vi "1_VisualAD_Train_Eval.vi"(0 "NNFE_Paths":T11={"CFG"=path "D:/Ngene/Projects_SVN/AD/Projects/2025/2025_04_09_VAD_RT_NIConnect/VAD_Host_Train_v1.0/NNFE/RN18_2/RN18_2_bnMerge.cfg", "BIN"=path "D:/Ngene/Projects_SVN/AD/Projects/2025/2025_04_09_VAD_RT_NIConnect/VAD_Host_Train_v1.0/NNFE/RN18_2/RN18_2_bnMerge.bin"}, 1 "Dest. Path":path=path "D:/Working/Cards_3Clubs", 2 "Dataset_Path(Train)":path=path "D:/DNN/_AD/_from_Customers/2025_04_12_NIConnect_3Clubs/1_Dataset/00_Orig/3Clubs/Train", 3 "Dataset_Path(Validation)":path=path "D:/DNN/_AD/_from_Customers/2025_04_12_NIConnect_3Clubs/1_Dataset/00_Orig/3Clubs/Test", 4 "Ground_Truth_Folder_Path":path, 5 "error in":errorcluster, 6 "NNFE_CFG":T7={"Name"="Cards_v2", "Layer_Selection_By"=enum."Layer_Idx", "Feature_Layers"={"[LayerID, PatchSize]"=[{"Layer_ID"=15, "Patch_Size"=5}]}, "Interpolation_Type"=enum."Bi-Linear"}, 7 "Dim_Reduction":T5={"Method"=enum."None", "Target_Dim"=-1, "Seed"=42}, 8 "NNPC_Setup":T13={"Input_Dims"={"C"=3, "H"=256, "W"=256}, "mBatch"=1, "Device"=enum."GPU", "GPU Id"=0}, 9 "Coreset_Params":T12={"CoreSet_Size"=1200.0, "Start_idx"=3}) -> (11 "MemBank Size":i32=1200, 13 "dT_Total":dbl=9.57656679999991 format="%.2p", 14 "NNPC_Paths":T11={"CFG"=path "D:/Working/Cards_3Clubs/NNPC_Cards_v2__25_04_14__17_27_09/NNPC_Cards_v2.cfg", "BIN"=path "D:/Working/Cards_3Clubs/NNPC_Cards_v2__25_04_14__17_27_09/NNPC_Cards_v2.bin"}, 15 "Evaluation_Metrics":T1={"Evaluation_Metrics(Pixel)"={"Scores(Good)"={"X Values"=[0.5210284759104251, 0.6102966575324535, 0.6995648391544819, 0.7888330207765102, 0.8781012023985386, 0.9673693840205669, 1.0566375656425953, 1.1459057472646235, 1.2351739288866521, 1.3244421105086803, 1.4137102921307085, 1.5029784737527372, 1.5922466553747654, 1.6815148369967936, 1.770783018618822, 1.8600512002408505, 1.9493193818628787, 2.0385875634849073, 2.1278557451069355, 2.2171239267289637, 2.306392108350992, 2.39566028997302, 2.484928471595049, 2.5741966532170775, 2.6634648348391057, 2.752733016461134, 2.842001198083162, 2.9312693797051903, 3.020537561327219, 3.109805742949247, 3.199073924571276, 3.288342106193304, 3.3776102878153322, 3.4668784694373604, 3.556146651059389, 3.6454148326814173, 3.734683014303446, 3.823951195925474, 3.9132193775475024, 4.002487559169531, 4.091755740791559, 4.181023922413587, 4.270292104035615, 4.359560285657643, 4.4488284672796725, 4.538096648901701, 4.627364830523729, 4.716633012145758, 4.805901193767786, 4.8951693753898144, 4.984437557011843, 5.073705738633871, 5.162973920255899, 5.252242101877927, 5.3415102834999555, 5.430778465121985, 5.520046646744013, 5.609314828366041, 5.698583009988069, 5.787851191610097, 5.8771193732321265, 5.966387554854155, 6.055655736476183, 6.144923918098211, 6.234192099720239, 6.323460281342268, 6.412728462964296, 6.501996644586324, 6.591264826208353, 6.680533007830381, 6.7698011894524095, 6.859069371074438, 6.948337552696466, 7.037605734318495, 7.126873915940523, 7.216142097562551, 7.30541027918458, 7.394678460806608, 7.483946642428636, 7.573214824050664, 7.6624830056726925, 7.751751187294722, 7.84101936891675, 7.930287550538778, 8.019555732160805, 8.108823913782834, 8.198092095404863, 8.287360277026892, 8.37662845864892, 8.465896640270948, 8.555164821892976, 8.644433003515005, 8.733701185137033, 8.822969366759061, 8.91223754838109, 9.001505730003117, 9.090773911625147, 9.180042093247176, 9.269310274869204, 9.358578456491232], "Histogram: h(x)"=[81, 124, 241, 366, 390, 655, 704, 909, 1257, 1569, 2363, 3876, 6095, 6433, 8148, 12170, 15948, 18555, 21356, 24301, 30533, 36030, 36647, 42002, 51965, 62635, 75376, 90060, 106995, 128101, 153148, 178169, 209892, 250937, 293012, 337008, 377469, 414170, 435302, 432424, 396009, 325877, 240699, 146788, 79579, 37092, 14124, 3355, 769, 100, 0, 0, 0, 0, 0, 0, 0, 0, 0, 0, 0, 0, 0, 0, 0, 0, 0, 0, 0, 0, 0, 0, 0, 0, 0, 0, 0, 0, 0, 0, 0, 0, 0, 0, 0, 0, 0, 0, 0, 0, 0, 0, 0, 0, 0, 0, 0, 0, 0, 0]}, "Scores(Bad)"={"X Values"=[0.5210284759104251, 0.6102966575324535, 0.6995648391544819, 0.7888330207765102, 0.8781012023985386, 0.9673693840205669, 1.0566375656425953, 1.1459057472646235, 1.2351739288866521, 1.3244421105086803, 1.4137102921307085, 1.5029784737527372, 1.5922466553747654, 1.6815148369967936, 1.770783018618822, 1.8600512002408505, 1.9493193818628787, 2.0385875634849073, 2.1278557451069355, 2.2171239267289637, 2.306392108350992, 2.39566028997302, 2.484928471595049, 2.5741966532170775, 2.6634648348391057, 2.752733016461134, 2.842001198083162, 2.9312693797051903, 3.020537561327219, 3.109805742949247, 3.199073924571276, 3.288342106193304, 3.3776102878153322, 3.4668784694373604, 3.556146651059389, 3.6454148326814173, 3.734683014303446, 3.823951195925474, 3.9132193775475024, 4.002487559169531, 4.091755740791559, 4.181023922413587, 4.270292104035615, 4.359560285657643, 4.4488284672796725, 4.538096648901701, 4.627364830523729, 4.716633012145758, 4.805901193767786, 4.8951693753898144, 4.984437557011843, 5.073705738633871, 5.162973920255899, 5.252242101877927, 5.3415102834999555, 5.430778465121985, 5.520046646744013, 5.609314828366041, 5.698583009988069, 5.787851191610097, 5.8771193732321265, 5.966387554854155, 6.055655736476183, 6.144923918098211, 6.234192099720239, 6.323460281342268, 6.412728462964296, 6.501996644586324, 6.591264826208353, 6.680533007830381, 6.7698011894524095, 6.859069371074438, 6.948337552696466, 7.037605734318495, 7.126873915940523, 7.216142097562551, 7.30541027918458, 7.394678460806608, 7.483946642428636, 7.573214824050664, 7.6624830056726925, 7.751751187294722, 7.84101936891675, 7.930287550538778, 8.019555732160805, 8.108823913782834, 8.198092095404863, 8.287360277026892, 8.37662845864892, 8.465896640270948, 8.555164821892976, 8.644433003515005, 8.733701185137033, 8.822969366759061, 8.91223754838109, 9.001505730003117, 9.090773911625147, 9.180042093247176, 9.269310274869204, 9.358578456491232], "Histogram: h(x)"=[131, 229, 343, 603, 652, 1004, 1224, 1485, 2177, 2667, 4288, 6774, 8552, 9591, 12914, 16677, 21984, 26086, 28236, 34100, 43533, 49702, 50940, 58577, 72709, 91728, 107407, 123475, 140133, 161571, 190960, 221005, 254784, 296306, 338720, 381955, 420647, 455243, 485230, 496593, 476018, 425984, 353689, 255448, 182116, 134329, 107803, 94493, 86226, 79961, 74940, 70797, 67724, 65255, 63380, 62473, 61758, 60556, 58820, 57829, 56854, 56149, 54719, 53459, 52357, 50751, 48587, 46892, 43031, 39688, 34785, 30380, 26158, 23541, 20915, 18284, 16302, 14200, 11400, 9383, 7280, 5316, 3813, 2689, 1681, 1310, 660, 301, 98, 55, 55, 53, 46, 44, 46, 37, 39, 36, 37, 35]}, "Eval Stats"={"Scores(Good)"={"Min"=0.49286556, "Max"=4.9073877}, "Scores(Bad)"={"Min"=0.4763944, "Max"=9.403213}, "# of Samples(Good)"=5111808, "# of Samples(Bad)"=8192000, "AUROC"=0.6164574, "F1_Max"=0.7621951, "Thrshld(F1_Max)"=0.4763944, "Prec.(F1_Max)"=0.61576355, "Recall(F1_Max)"=1.0, "FPR(F1_Max)"=1.0, "FNR(F1_Max)"=0.0}}, "Evaluation_Metrics(Image)"={"Scores(Good)"={"X Values"=[4.919271998405456, 4.968675293922424, 5.0180785894393924, 5.06748188495636, 5.116885180473328, 5.166288475990296, 5.215691771507263, 5.26509506702423, 5.314498362541199, 5.363901658058166, 5.413304953575134, 5.462708249092103, 5.51211154460907, 5.561514840126037, 5.610918135643006, 5.660321431159973, 5.70972472667694, 5.759128022193909, 5.808531317710877, 5.857934613227844, 5.907337908744813, 5.95674120426178, 6.006144499778747, 6.055547795295716, 6.104951090812683, 6.154354386329651, 6.203757681846619, 6.253160977363587, 6.302564272880554, 6.351967568397521, 6.40137086391449, 6.450774159431457, 6.500177454948425, 6.549580750465394, 6.598984045982361, 6.648387341499328, 6.697790637016297, 6.747193932533264, 6.796597228050231, 6.8460005235672, 6.8954038190841676, 6.944807114601135, 6.994210410118104, 7.043613705635071, 7.093017001152038, 7.142420296669007, 7.191823592185974, 7.2412268877029415, 7.2906301832199105, 7.340033478736878, 7.389436774253845, 7.438840069770813, 7.488243365287781, 7.537646660804748, 7.5870499563217155, 7.6364532518386845, 7.685856547355652, 7.735259842872619, 7.784663138389588, 7.834066433906555, 7.883469729423522, 7.932873024940491, 7.9822763204574585, 8.031679615974426, 8.081082911491393, 8.130486207008362, 8.17988950252533, 8.229292798042298, 8.278696093559265, 8.328099389076232, 8.3775026845932, 8.426905980110169, 8.476309275627138, 8.525712571144105, 8.575115866661072, 8.62451916217804, 8.673922457695006, 8.723325753211975, 8.772729048728943, 8.822132344245912, 8.871535639762879, 8.920938935279846, 8.970342230796813, 9.01974552631378, 9.06914882183075, 9.118552117347718, 9.167955412864686, 9.217358708381653, 9.26676200389862, 9.316165299415587, 9.365568594932556, 9.414971890449525, 9.464375185966492, 9.51377848148346, 9.563181777000427, 9.612585072517394, 9.661988368034363, 9.711391663551332, 9.7607949590683, 9.810198254585266], "Histogram: h(x)"=[3, 4, 10, 14, 14, 14, 9, 4, 3, 2, 0, 0, 0, 1, 0, 0, 0, 0, 0, 0, 0, 0, 0, 0, 0, 0, 0, 0, 0, 0, 0, 0, 0, 0, 0, 0, 0, 0, 0, 0, 0, 0, 0, 0, 0, 0, 0, 0, 0, 0, 0, 0, 0, 0, 0, 0, 0, 0, 0, 0, 0, 0, 0, 0, 0, 0, 0, 0, 0, 0, 0, 0, 0, 0, 0, 0, 0, 0, 0, 0, 0, 0, 0, 0, 0, 0, 0, 0, 0, 0, 0, 0, 0, 0, 0, 0, 0, 0, 0, 0]}, "Scores(Bad)"={"X Values"=[4.919271998405456, 4.968675293922424, 5.0180785894393924, 5.06748188495636, 5.116885180473328, 5.166288475990296, 5.215691771507263, 5.26509506702423, 5.314498362541199, 5.363901658058166, 5.413304953575134, 5.462708249092103, 5.51211154460907, 5.561514840126037, 5.610918135643006, 5.660321431159973, 5.70972472667694, 5.759128022193909, 5.808531317710877, 5.857934613227844, 5.907337908744813, 5.95674120426178, 6.006144499778747, 6.055547795295716, 6.104951090812683, 6.154354386329651, 6.203757681846619, 6.253160977363587, 6.302564272880554, 6.351967568397521, 6.40137086391449, 6.450774159431457, 6.500177454948425, 6.549580750465394, 6.598984045982361, 6.648387341499328, 6.697790637016297, 6.747193932533264, 6.796597228050231, 6.8460005235672, 6.8954038190841676, 6.944807114601135, 6.994210410118104, 7.043613705635071, 7.093017001152038, 7.142420296669007, 7.191823592185974, 7.2412268877029415, 7.2906301832199105, 7.340033478736878, 7.389436774253845, 7.438840069770813, 7.488243365287781, 7.537646660804748, 7.5870499563217155, 7.6364532518386845, 7.685856547355652, 7.735259842872619, 7.784663138389588, 7.834066433906555, 7.883469729423522, 7.932873024940491, 7.9822763204574585, 8.031679615974426, 8.081082911491393, 8.130486207008362, 8.17988950252533, 8.229292798042298, 8.278696093559265, 8.328099389076232, 8.3775026845932, 8.426905980110169, 8.476309275627138, 8.525712571144105, 8.575115866661072, 8.62451916217804, 8.673922457695006, 8.723325753211975, 8.772729048728943, 8.822132344245912, 8.871535639762879, 8.920938935279846, 8.970342230796813, 9.01974552631378, 9.06914882183075, 9.118552117347718, 9.167955412864686, 9.217358708381653, 9.26676200389862, 9.316165299415587, 9.365568594932556, 9.414971890449525, 9.464375185966492, 9.51377848148346, 9.563181777000427, 9.612585072517394, 9.661988368034363, 9.711391663551332, 9.7607949590683, 9.810198254585266], "Histogram: h(x)"=[0, 0, 0, 0, 0, 0, 0, 0, 0, 0, 0, 0, 0, 0, 0, 0, 0, 0, 0, 0, 0, 0, 0, 0, 0, 0, 0, 0, 0, 4, 0, 2, 1, 3, 6, 6, 6, 7, 1, 1, 6, 3, 0, 2, 0, 0, 1, 0, 0, 1, 1, 2, 0, 2, 2, 0, 0, 1, 0, 0, 3, 6, 5, 5, 2, 5, 5, 8, 4, 6, 2, 4, 4, 0, 4, 2, 0, 0, 1, 0, 0, 0, 0, 0, 0, 0, 0, 0, 0, 0, 0, 0, 0, 0, 0, 0, 0, 0, 0, 1]}, "Eval Stats"={"Scores(Good)"={"Min"=4.8945704, "Max"=5.5621405}, "Scores(Bad)"={"Min"=6.3359256, "Max"=9.8349}, "# of Samples(Good)"=78, "# of Samples(Bad)"=125, "AUROC"=1.0, "F1_Max"=1.0, "Thrshld(F1_Max)"=5.5621824, "Prec.(F1_Max)"=1.0, "Recall(F1_Max)"=1.0, "FPR(F1_Max)"=0.0, "FNR(F1_Max)"=0.0}}} {"Evaluation_Metrics(Image)"."Eval Stats"."Recall(F1_Max)" format="%#.5f"; "Evaluation_Metrics(Image)"."Eval Stats"."FPR(F1_Max)" format="%#.5f"; "Evaluation_Metrics(Image)"."Eval Stats"."FNR(F1_Max)" format="%#.5f"; "Evaluation_Metrics(Image)"."Eval Stats"."Prec.(F1_Max)" format="%#.5f"; "Evaluation_Metrics(Image)"."Eval Stats"."F1_Max" format="%#.5f"; "Evaluation_Metrics(Image)"."Eval Stats"."AUROC" format="%#.5f"; "Evaluation_Metrics(Image)"."Eval Stats"."Scores(Bad)"."Min" format="%#_5g"; "Evaluation_Metrics(Image)"."Eval Stats"."Scores(Good)"."Min" format="%#_5g"; "Evaluation_Metrics(Image)"."Eval Stats"."Thrshld(F1_Max)" format="%#_5f"; "Evaluation_Metrics(Pixel)"."Eval Stats"."Recall(F1_Max)" format="%#.5f"; "Evaluation_Metrics(Pixel)"."Eval Stats"."FPR(F1_Max)" format="%#.5f"; "Evaluation_Metrics(Pixel)"."Eval Stats"."FNR(F1_Max)" format="%#.5f"; "Evaluation_Metrics(Pixel)"."Eval Stats"."Prec.(F1_Max)" format="%#.5f"; "Evaluation_Metrics(Pixel)"."Eval Stats"."F1_Max" format="%#.5f"; "Evaluation_Metrics(Pixel)"."Eval Stats"."AUROC" format="%#.5f"; "Evaluation_Metrics(Pixel)"."Eval Stats"."Scores(Bad)"."Min" format="%#_5g"; "Evaluation_Metrics(Pixel)"."Eval Stats"."Scores(Good)"."Min" format="%#_5g"; "Evaluation_Metrics(Pixel)"."Eval Stats"."Thrshld(F1_Max)" format="%#_5f"}, 18 "Dataset Size":i32=285)   [LabVIEW 2020]
uses:
  <vilib>/Ngene/DeepLTK Anomaly Detection Addon/DeepLTK_Anomaly_Detection_Addon/API/Controls/NN_Paths.ctl
  <vilib>/Ngene/DeepLTK Anomaly Detection Addon/DeepLTK_Anomaly_Detection_Addon/API/Controls/NNPC_Setup.ctl
  <vilib>/Ngene/Deep Learning Toolkit/Toolkit/NN_Data/API/NN_Dims(C,H,W).ctl
  <vilib>/Ngene/Deep Learning Toolkit/Toolkit/NN_Network/Controls/NN_Device.ctl
  <vilib>/Ngene/DeepLTK Anomaly Detection Addon/DeepLTK_Anomaly_Detection_Addon/API/Controls/NNPC_Coreset_Params.ctl
  <vilib>/Ngene/DeepLTK Anomaly Detection Addon/DeepLTK_Anomaly_Detection_Addon/API/Controls/NNFE_CFG.ctl
  <vilib>/Ngene/DeepLTK Anomaly Detection Addon/DeepLTK_Anomaly_Detection_Addon/API/Controls/Layer_Selector.ctl
  <vilib>/Ngene/DeepLTK Anomaly Detection Addon/DeepLTK_Anomaly_Detection_Addon/API/Controls/Feature_Layer_Selector.ctl
  <vilib>/Ngene/DeepLTK Anomaly Detection Addon/DeepLTK_Anomaly_Detection_Addon/API/Controls/Interpolation_Selector.ctl
  <vilib>/Ngene/DeepLTK Anomaly Detection Addon/DeepLTK_Anomaly_Detection_Addon/API/Controls/NNPC_Random_Projection_CFG.ctl
  <vilib>/Ngene/DeepLTK Anomaly Detection Addon/DeepLTK_Anomaly_Detection_Addon/API/Controls/Dim_Reduction_Method.ctl
  <vilib>/Ngene/DeepLTK Anomaly Detection Addon/DeepLTK_Anomaly_Detection_Addon/API/Controls/Evaluation_Metrics(Pixel_Image).ctl
  <vilib>/Ngene/DeepLTK Anomaly Detection Addon/DeepLTK_Anomaly_Detection_Addon/API/Controls/Evaluation_Metrics.ctl
  <vilib>/Ngene/DeepLTK Anomaly Detection Addon/DeepLTK_Anomaly_Detection_Addon/API/Controls/Eval_Results.ctl
  <vilib>/Ngene/DeepLTK Anomaly Detection Addon/DeepLTK_Anomaly_Detection_Addon/API/Controls/MinMax.ctl
  <vilib>/Ngene/DeepLTK Anomaly Detection Addon/DeepLTK_Anomaly_Detection_Addon/API/Controls/NNPC_Save_CFG.ctl
  <vilib>/Ngene/DeepLTK Anomaly Detection Addon/DeepLTK_Anomaly_Detection_Addon/API/Controls/NNPC_PreProcessing_Options.ctl
  <vilib>/Ngene/DeepLTK Anomaly Detection Addon/DeepLTK_Anomaly_Detection_Addon/API/Controls/NNPC_DS_Stats.ctl
  <vilib>/Ngene/DeepLTK Anomaly Detection Addon/DeepLTK_Anomaly_Detection_Addon/API/Controls/Image_Stats_RGB.ctl
  subVIs/Dataset_Reader/Controls/Read_Options.ctl
  <vilib>/Ngene/DeepLTK Anomaly Detection Addon/DeepLTK_Anomaly_Detection_Addon/API/NNPC_Generate_Embedding/NNPC_Generate_Embedding(Dataset).vi
  <vilib>/Ngene/DeepLTK Anomaly Detection Addon/DeepLTK_Anomaly_Detection_Addon/API/NNPC_Predict/NNPC_Predict(Dataset).vi
  <vilib>/Ngene/Deep Learning Toolkit/Toolkit/NN_Data/subVIs/Dataset_Destroy/NN_Dataset_Destroy(In3D_Out3D).vi
  <vilib>/Ngene/Deep Learning Toolkit/Toolkit/Deep_Learning_Toolkit_by_Ngene.lvlib
  <vilib>/Ngene/DeepLTK Anomaly Detection Addon/DeepLTK_Anomaly_Detection_Addon/DeepLTK_Anomaly_Detection_Addon.lvlib
panel:
  out "Feature Size":i32=128
  out "error out":errorcluster
  out "Coreset Min":sgl=5.160844
  out "Coreset Max":sgl=19.46937
  out "dT_Predict":dbl=0.5213928000000578 format="%.2p"
  out "dT_Eval":dbl=3.1058166000000256 format="%.2p"
  out "dT_Read_DS(Test)":dbl=2.2328044000000773 format="%.2p"
  out "dT_Read_DS(Train)":dbl=3.5484586999998555 format="%.2p"
  out "dT_NN_Init":dbl=0.5681460999999217 format="%.2p"
  out "Coreset_Max_Distances":sgl[](graph)=[19.46937, 16.781397, 14.001281, 13.836462, 13.739045, 13.200295, 13.1346245, 12.7480755, 12.133151, 11.688953, 11.562293, 11.521474, 11.431094, 11.274108, 11.229277, 11.169556, 11.083287, 10.935635, 10.858421, 10.807946, 10.589487, 10.50305, 10.480584, 10.4153595, 10.357788, 10.130338, 10.12428, 10.081089, 10.0776615, 9.983067, 9.924832, 9.915435, 9.884131, 9.870699, 9.85285, 9.725132, 9.696888, 9.675768, 9.64603, 9.645999, 9.541911, 9.518525, 9.453406, 9.437411, 9.435752, 9.389733, 9.381479, 9.36939, 9.320507, 9.282261, 9.261716, 9.232438, 9.134313, 9.117022, 9.116268, 9.044784, 9.028286, 9.010026, 8.983074, 8.971089, 8.858672, 8.845759, 8.840825, 8.830351, 8.809639, 8.80413, 8.781888, 8.748896, 8.719765, 8.715809, 8.696731, 8.6775675, 8.667834, 8.641909, 8.6257515, 8.603801, 8.565515, 8.5644455, 8.549131, 8.536594, 8.514139, 8.488552, 8.475194, 8.468653, 8.454728, 8.427404, 8.376778, 8.365597, 8.351924, 8.348353, 8.339942, 8.325125, 8.303677, 8.291491, 8.268808, 8.260227, 8.25838, 8.234027, 8.224351, 8.217981, 8.205, 8.191266, 8.13027, 8.124921, 8.121136, 8.108029, 8.091195, 8.082535, 8.079678, 8.071409, 8.068754, 8.062763, 8.04005, 8.0156765, 7.9833508, 7.9817734, 7.9756866, 7.9674706, 7.955339, 7.954186, 7.9532056, 7.951235, 7.932406, 7.9036345, 7.8951316, 7.894743, 7.884721, 7.8842, 7.861708, 7.843711, 7.8291306, 7.8041654, 7.802609, 7.7963605, 7.7932577, 7.787836, 7.777994, 7.768069, 7.76735, 7.7649727, 7.7557883, 7.742485, 7.72457, 7.720849, 7.720424, 7.7061787, 7.6922684, 7.654444, 7.653362, 7.645953, 7.6325245, 7.623823, 7.6200075, 7.597344, 7.591033, 7.5791984, 7.575896, 7.573134, 7.5683107, 7.567111, 7.5648885, 7.5555177, 7.5493193, 7.5422254, 7.5120873, 7.502437, 7.500528, 7.4817066, 7.477346, 7.4752254, 7.4747458, 7.4741282, 7.4712133, 7.455745, 7.446993, 7.443767, 7.4243193, 7.4176674, 7.416217, 7.4160852, 7.4139676, 7.4089565, 7.4084272, 7.399413, 7.3951864, 7.3940825, 7.3912115, 7.389731, 7.368076, 7.3674774, 7.3668766, 7.363222, 7.3573623, 7.337048, 7.3313246, 7.325255, 7.324968, 7.323693, 7.3220134, 7.3206563, 7.3185635, 7.318065, 7.303977, 7.291284, 7.279843, 7.2771497, 7.2746754, 7.246301, 7.2461243, 7.243245, 7.242394, 7.2367034, 7.2228603, 7.214697, 7.2118196, 7.206732, 7.18588, 7.176505, 7.1760736, 7.1721196, 7.1578617, 7.1497097, 7.146749, 7.1445727, 7.1393065, 7.1373143, 7.136985, 7.1265244, 7.1151376, 7.1098557, 7.107177, 7.089042, 7.087757, 7.086635, 7.0733504, 7.072466, 7.062424, 7.054523, 7.053416, 7.051845, 7.0364347, 7.034743, 7.029583, 7.02008, 7.014531, 7.0104465, 7.0066824, 7.005759, 7.005667, 7.0022926, 6.9957547, 6.994208, 6.987603, 6.984908, 6.978115, 6.9691133, 6.9688706, 6.9617443, 6.9612446, 6.944324, 6.942715, 6.9325075, 6.923096, 6.905236, 6.9001384, 6.899265, 6.8963866, 6.8704596, 6.869638, 6.869458, 6.863222, 6.861132, 6.850164, 6.8474054, 6.8398046, 6.831105, 6.82602, 6.82428, 6.814876, 6.8023686, 6.7976675, 6.7915907, 6.790449, 6.788597, 6.783666, 6.777097, 6.7768, 6.7766695, 6.7756424, 6.7756314, 6.7743025, 6.7706504, 6.769866, 6.7661753, 6.7629337, 6.7596316, 6.7594075, 6.7484965, 6.7453437, 6.7376823, 6.731993, 6.727994, 6.724348, 6.7240124, 6.718407, 6.7123427, 6.7033186, 6.7010183, 6.700698, 6.6960373, 6.692671, 6.6923537, 6.6918955, 6.691252, 6.6697273, 6.665576, 6.665223, 6.660309, 6.6597266, 6.659044, 6.6538057, 6.6527185, 6.6511774, 6.6489587, 6.640832, 6.6406984, 6.6404, 6.636598, 6.629583, 6.6145883, 6.611282, 6.609181, 6.6089616, 6.6086326, 6.6038976, 6.5997596, 6.5987697, 6.590461, 6.5878315, 6.586118, 6.585808, 6.5830593, 6.581154, 6.577355, 6.576863, 6.576478, 6.57616, 6.5730104, 6.5719056, 6.5660796, 6.565064, 6.561449, 6.557769, 6.5516324, 6.5426483, 6.5376134, 6.5357857, 6.5316052, 6.5263653, 6.521498, 6.5108414, 6.5060773, 6.505716, 6.502103, 6.500216, 6.498325, 6.4902883, 6.4879932, 6.4849396, 6.4795256, 6.478878, 6.473216, 6.472332, 6.471974, 6.458823, 6.4584785, 6.458313, 6.4524345, 6.4481573, 6.4459114, 6.444943, 6.441784, 6.435836, 6.435274, 6.433396, 6.4295144, 6.427682, 6.4266396, 6.4229894, 6.4196053, 6.40881, 6.406805, 6.4055495, 6.403603, 6.3955894, 6.389062, 6.377372, 6.3744783, 6.3712792, 6.3692875, 6.368519, 6.3667226, 6.3636675, 6.361016, 6.3589673, 6.355669, 6.3507648, 6.3488026, 6.347823, 6.3443103, 6.3408823, 6.330032, 6.3298054, 6.329122, 6.328764, 6.3273993, 6.326635, 6.3226686, 6.319564, 6.31388, 6.303194, 6.297246, 6.2956243, 6.2950864, 6.2939253, 6.2923446, 6.290736, 6.2880774, 6.286995, 6.2822704, 6.279265, 6.279068, 6.2788982, 6.2747655, 6.2739897, 6.2689447, 6.2689238, 6.26832, 6.266219, 6.2640443, 6.2632647, 6.263146, 6.259692, 6.257132, 6.2538624, 6.246298, 6.2423954, 6.240452, 6.235743, 6.235246, 6.2324266, 6.231719, 6.2301493, 6.229407, 6.2281036, 6.2278147, 6.22595, 6.224874, 6.2246947, 6.224668, 6.2191525, 6.2155495, 6.203575, 6.200505, 6.1944675, 6.194056, 6.1930065, 6.1901145, 6.189842, 6.1894703, 6.183918, 6.1834593, 6.1829906, 6.181075, 6.176697, 6.170592, 6.169986, 6.167898, 6.167234, 6.1663346, 6.165869, 6.161, 6.1559253, 6.1555114, 6.1534534, 6.1515837, 6.1507354, 6.1460795, 6.143158, 6.1425877, 6.141204, 6.1399193, 6.1362004, 6.132127, 6.131409, 6.126009, 6.124305, 6.1242175, 6.1213865, 6.1176915, 6.1158905, 6.1138315, 6.1086206, 6.106722, 6.10558, 6.103378, 6.1004343, 6.0974236, 6.0928483, 6.0897675, 6.0888, 6.087118, 6.08684, 6.0852604, 6.0849895, 6.07245, 6.0723405, 6.0687084, 6.066394, 6.065605, 6.0629683, 6.061, 6.060224, 6.0553074, 6.0544405, 6.050914, 6.048109, 6.0468297, 6.0451436, 6.042859, 6.042392, 6.0418816, 6.0381856, 6.0340776, 6.0311866, 6.0307817, 6.0263476, 6.025347, 6.0250516, 6.02304, 6.020529, 6.0193653, 6.018027, 6.017943, 6.0176616, 6.017152, 6.0130625, 6.012938, 6.0117455, 6.0101027, 6.009872, 6.0041666, 6.0019784, 5.999494, 5.999377, 5.9982476, 5.9939876, 5.993504, 5.993242, 5.989355, 5.9884253, 5.986374, 5.9857235, 5.984439, 5.9827213, 5.980404, 5.9795976, 5.976629, 5.9749255, 5.9734697, 5.9721336, 5.96964, 5.9592915, 5.9525895, 5.952138, 5.9515867, 5.951043, 5.947568, 5.9464903, 5.946198, 5.941341, 5.9401107, 5.9390826, 5.936706, 5.935441, 5.9347935, 5.9280095, 5.925126, 5.920848, 5.9207153, 5.916531, 5.9163404, 5.915556, 5.9146585, 5.9138327, 5.9130535, 5.910222, 5.9045057, 5.9031854, 5.8994384, 5.895014, 5.8940253, 5.893919, 5.893867, 5.8931036, 5.8903713, 5.889797, 5.8846745, 5.8827477, 5.8799067, 5.877594, 5.8766932, 5.8763866, 5.8741426, 5.873964, 5.8717837, 5.8711367, 5.870796, 5.870531, 5.8704295, 5.8687296, 5.8669195, 5.86463, 5.8642063, 5.863202, 5.8621244, 5.8610153, 5.8599296, 5.8545265, 5.853346, 5.851286, 5.851114, 5.8509655, 5.849069, 5.847587, 5.8467574, 5.844426, 5.8401914, 5.8379674, 5.837177, 5.8345413, 5.8321767, 5.831978, 5.8268733, 5.8257866, 5.8257837, 5.8241625, 5.818785, 5.817719, 5.8165307, 5.8157387, 5.812503, 5.811815, 5.810423, 5.8098845, 5.808364, 5.807289, 5.805923, 5.8028154, 5.8026104, 5.8017297, 5.8012137, 5.7984543, 5.7933073, 5.791263, 5.791155, 5.790459, 5.7901406, 5.788712, 5.788314, 5.787552, 5.7867503, 5.779917, 5.773319, 5.770048, 5.7696013, 5.768948, 5.7677007, 5.762133, 5.7616405, 5.7615905, 5.7615294, 5.7609706, 5.7593203, 5.7554693, 5.7545877, 5.753844, 5.7533507, 5.7521462, 5.7520046, 5.750407, 5.749549, 5.7477174, 5.7475767, 5.7463155, 5.7428465, 5.7367134, 5.7366924, 5.7353196, 5.7340755, 5.7284913, 5.728113, 5.72628, 5.7242627, 5.722196, 5.7220445, 5.720249, 5.719006, 5.7176213, 5.717117, 5.7134967, 5.7116714, 5.711202, 5.707586, 5.70703, 5.7045107, 5.7038927, 5.702761, 5.701672, 5.700588, 5.6996083, 5.695468, 5.69321, 5.6920295, 5.69174, 5.6905065, 5.6885033, 5.688321, 5.6876287, 5.6867566, 5.6865716, 5.6854153, 5.6822286, 5.6810412, 5.680413, 5.679663, 5.677132, 5.676949, 5.676597, 5.6726522, 5.6726513, 5.670344, 5.669873, 5.667197, 5.6662483, 5.66518, 5.6647468, 5.6629066, 5.658427, 5.6578574, 5.651535, 5.6494746, 5.6440597, 5.643535, 5.64271, 5.641968, 5.6402936, 5.638739, 5.638501, 5.636824, 5.635881, 5.634294, 5.6340313, 5.633896, 5.630523, 5.629753, 5.628536, 5.626306, 5.621939, 5.617637, 5.6176357, 5.6157746, 5.6138587, 5.6119475, 5.610047, 5.6098757, 5.607039, 5.606956, 5.606341, 5.6043773, 5.601486, 5.6014347, 5.600933, 5.5993557, 5.5984564, 5.597404, 5.5973196, 5.5960274, 5.595003, 5.593165, 5.5924597, 5.592001, 5.5914826, 5.588947, 5.5870547, 5.586424, 5.5848584, 5.584386, 5.5831614, 5.5804796, 5.5795336, 5.57786, 5.5774164, 5.5768228, 5.575394, 5.57468, 5.572427, 5.5718737, 5.571682, 5.567345, 5.5658183, 5.5647597, 5.5592074, 5.5588613, 5.558171, 5.557966, 5.5578074, 5.5572968, 5.556923, 5.5542097, 5.553869, 5.5524483, 5.548146, 5.547953, 5.5469356, 5.543694, 5.5428805, 5.542075, 5.541819, 5.5410013, 5.5403404, 5.5391026, 5.5371337, 5.5370374, 5.536503, 5.533594, 5.53296, 5.52891, 5.528253, 5.5187116, 5.518678, 5.5182137, 5.518098, 5.517298, 5.516051, 5.514759, 5.513331, 5.5133104, 5.5108204, 5.5098734, 5.5090036, 5.5088234, 5.508699, 5.508566, 5.5081477, 5.507203, 5.506516, 5.5062165, 5.5057344, 5.5048723, 5.5035777, 5.50218, 5.5015063, 5.500548, 5.500391, 5.500197, 5.498979, 5.498929, 5.4988847, 5.497608, 5.494467, 5.49396, 5.493846, 5.492718, 5.491132, 5.491118, 5.4894195, 5.4882407, 5.4862914, 5.4855127, 5.484606, 5.484247, 5.481052, 5.4773564, 5.4771366, 5.4747095, 5.4732404, 5.472981, 5.4728613, 5.470265, 5.468648, 5.4671593, 5.467094, 5.4656773, 5.465163, 5.464834, 5.464468, 5.4642086, 5.462583, 5.458433, 5.4572873, 5.4562244, 5.455945, 5.4535193, 5.4528255, 5.4523444, 5.449699, 5.4492846, 5.448845, 5.443003, 5.44205, 5.4409156, 5.4398565, 5.439349, 5.4393125, 5.4391975, 5.4385777, 5.438314, 5.4347157, 5.4332848, 5.432466, 5.4318957, 5.4308844, 5.428993, 5.4285603, 5.4285197, 5.4283214, 5.4268484, 5.425153, 5.423749, 5.4216247, 5.421453, 5.4210477, 5.42098, 5.420752, 5.419726, 5.418705, 5.4177423, 5.4170885, 5.4167476, 5.416542, 5.4147387, 5.4144654, 5.4125543, 5.412284, 5.4097486, 5.409111, 5.408815, 5.4068737, 5.40472, 5.403407, 5.402924, 5.4018564, 5.400738, 5.3998733, 5.39874, 5.398344, 5.3981633, 5.3977957, 5.395879, 5.395684, 5.393079, 5.392438, 5.3905287, 5.3903704, 5.3895974, 5.386573, 5.3863916, 5.3862243, 5.3861876, 5.385176, 5.3817835, 5.381004, 5.379509, 5.378746, 5.3777475, 5.3776765, 5.3764563, 5.3760786, 5.37582, 5.3750596, 5.3732085, 5.372291, 5.371689, 5.370734, 5.369484, 5.36806, 5.365658, 5.3652883, 5.365132, 5.3650603, 5.363351, 5.360827, 5.3606334, 5.3588114, 5.3570485, 5.35606, 5.353849, 5.352777, 5.351748, 5.3491325, 5.3489614, 5.34822, 5.343313, 5.3428974, 5.342545, 5.3421793, 5.3416367, 5.341528, 5.341448, 5.341411, 5.341228, 5.3409796, 5.339614, 5.339405, 5.3384104, 5.337047, 5.3367496, 5.3362923, 5.33517, 5.334908, 5.3344245, 5.333569, 5.3318496, 5.3299503, 5.3278527, 5.3277025, 5.3253293, 5.3220587, 5.3209577, 5.3203926, 5.318723, 5.3185887, 5.318465, 5.316158, 5.315231, 5.3149266, 5.314542, 5.312463, 5.312443, 5.3115406, 5.3083854, 5.3064117, 5.3051705, 5.3047423, 5.303301, 5.3024664, 5.300941, 5.2952213, 5.2951407, 5.2948523, 5.294426, 5.292336, 5.291635, 5.2915745, 5.2901154, 5.2893395, 5.2887135, 5.288415, 5.2880006, 5.2874465, 5.286901, 5.285946, 5.2851143, 5.2845774, 5.2805796, 5.2800927, 5.280022, 5.279288, 5.27668, 5.2746644, 5.2746005, 5.2734866, 5.273229, 5.273099, 5.2729716, 5.272584, 5.2721295, 5.2680936, 5.2676764, 5.2665596, 5.2650075, 5.264802, 5.2640367, 5.2627206, 5.260482, 5.2602205, 5.259733, 5.256939, 5.2557282, 5.255043, 5.254666, 5.2506247, 5.249279, 5.2481103, 5.2474184, 5.2472525, 5.247055, 5.246098, 5.2455006, 5.244719, 5.2446117, 5.243148, 5.242352, 5.241218, 5.240221, 5.2390895, 5.23807, 5.237508, 5.2374525, 5.2372136, 5.23594, 5.2355266, 5.235465, 5.235092, 5.2348995, 5.2345967, 5.234524, 5.229344, 5.229122, 5.2287283, 5.22867, 5.2283926, 5.227425, 5.2269683, 5.226297, 5.2244163, 5.2233386, 5.221898, 5.221825, 5.2177205, 5.217542, 5.216659, 5.2166123, 5.2163053, 5.2143593, 5.213069, 5.213025, 5.2126822, 5.212375, 5.2120824, 5.211538, 5.2108088, 5.210683, 5.2091303, 5.2059484, 5.2057753, 5.2046704, 5.2041893, 5.204096, 5.2039504, 5.2034593, 5.203043, 5.2016206, 5.201069, 5.199408, 5.198249, 5.1980786, 5.1979814, 5.1976995, 5.1966224, 5.196337, 5.1951747, 5.1940026, 5.1939964, 5.1939435, 5.192448, 5.1919928, 5.1908755, 5.1900554, 5.1895294, 5.185629, 5.1853642, 5.183059, 5.1830153, 5.182933, 5.182191, 5.181465, 5.1810985, 5.1804595, 5.1793075, 5.179026, 5.178014, 5.1779094, 5.174323, 5.1742187, 5.1721716, 5.170739, 5.169626, 5.169358, 5.168735, 5.1682906, 5.16748, 5.1673517, 5.166299, 5.164863, 5.164813, 5.163362, 5.1621976, 5.160844]
  out "dT_Coreset":dbl=0.5992286999999124 format="%.2p"
  out "dT_Gen_Embed":dbl=0.7023947000000135 format="%.2p"
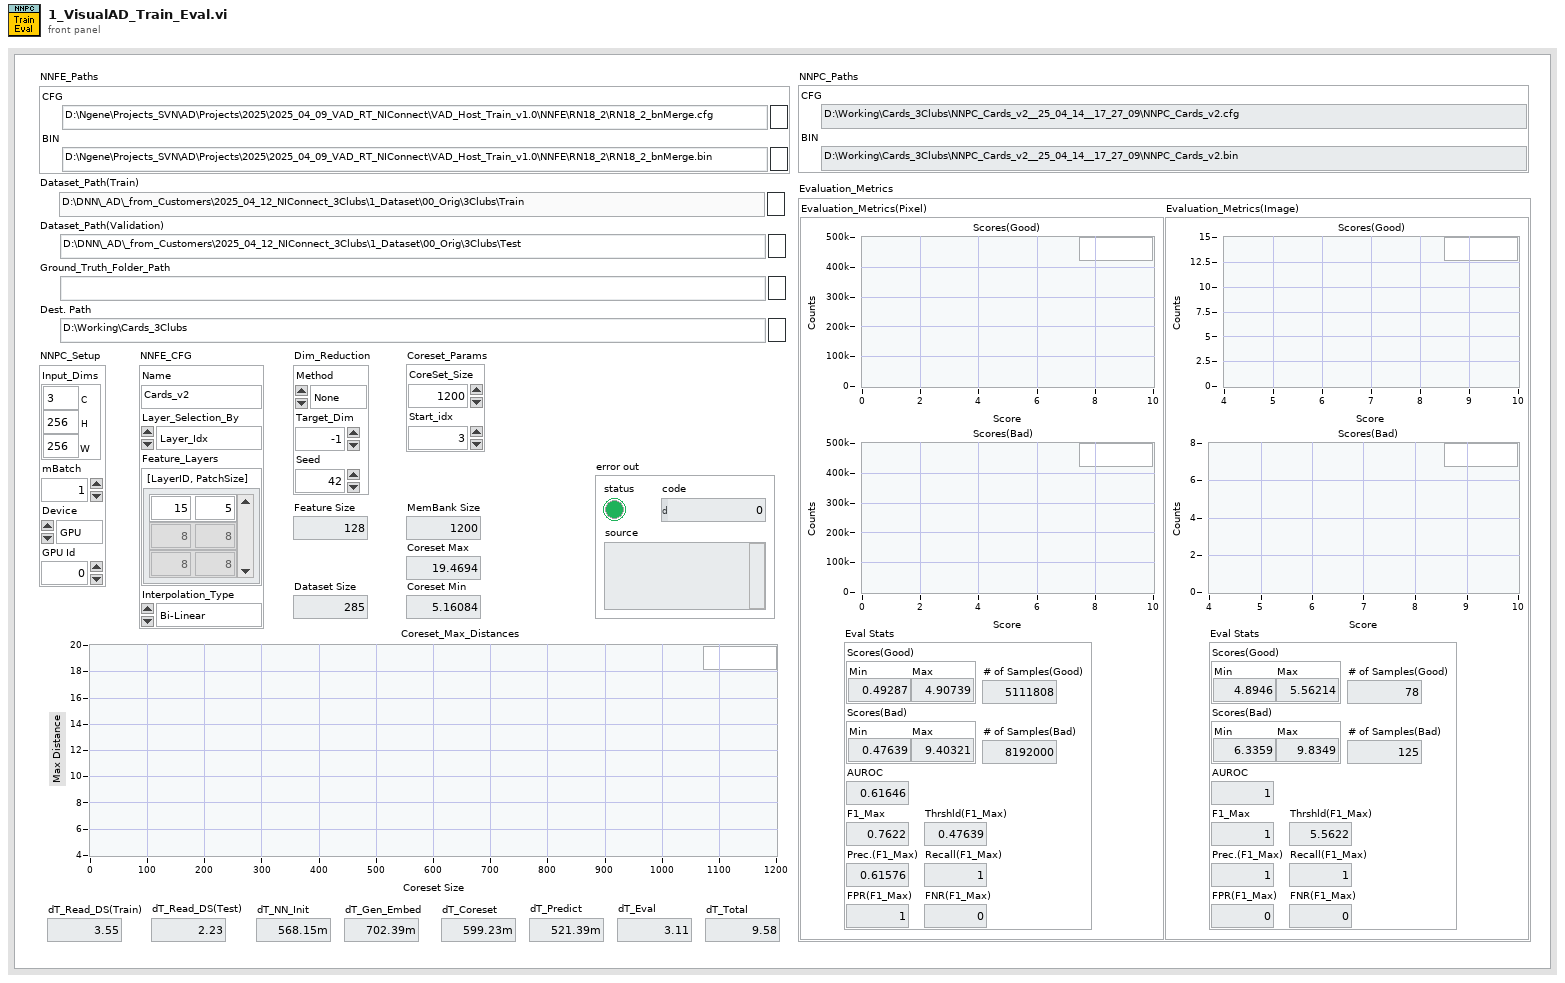
[diagram p1: front panel]
types:
  T1 = typedef "DeepLTK_Anomaly_Detection_Addon.lvlib/Evaluation_Metrics(Pixel_Image).ctl" = cluster{"Evaluation_Metrics(Pixel)":T2, "Evaluation_Metrics(Image)":T2}
  T2 = typedef "DeepLTK_Anomaly_Detection_Addon.lvlib/Evaluation_Metrics.ctl" = cluster{"Scores(Good)":cluster{"X Values":dbl[], "Histogram: h(x)":i32[]}, "Scores(Bad)":cluster{"X Values":dbl[], "Histogram: h(x)":i32[]}, "Eval Stats":T3}
  T3 = typedef "DeepLTK_Anomaly_Detection_Addon.lvlib/Eval_Results.ctl" = cluster{"Scores(Good)":T4, "Scores(Bad)":T4, "# of Samples(Good)":i32, "# of Samples(Bad)":i32, "AUROC":sgl, "F1_Max":sgl, "Thrshld(F1_Max)":sgl, "Prec.(F1_Max)":sgl, "Recall(F1_Max)":sgl, "FPR(F1_Max)":sgl, "FNR(F1_Max)":sgl}
  T4 = typedef "DeepLTK_Anomaly_Detection_Addon.lvlib/MinMax.ctl" = cluster{"Min":sgl, "Max":sgl}
  T5 = typedef "DeepLTK_Anomaly_Detection_Addon.lvlib/NNPC_Random_Projection_CFG.ctl" = cluster{"Method":T6, "Target_Dim":i32, "Seed":i32}
  T6 = typedef "DeepLTK_Anomaly_Detection_Addon.lvlib/Dim_Reduction_Method.ctl" = enum16{"None", "Rnd_Proj", "PCA"}
  T7 = typedef "DeepLTK_Anomaly_Detection_Addon.lvlib/NNFE_CFG.ctl" = cluster{"Name":string, "Layer_Selection_By":T8, "Feature_Layers":T9, "Interpolation_Type":T10}
  T8 = typedef "DeepLTK_Anomaly_Detection_Addon.lvlib/Layer_Selector.ctl" = enum16{"Stride", "Layer_Idx"}
  T9 = typedef "DeepLTK_Anomaly_Detection_Addon.lvlib/Feature_Layer_Selector.ctl" = cluster{"[LayerID, PatchSize]":cluster{"Layer_ID":i32, "Patch_Size":i32}[]}
  T10 = typedef "DeepLTK_Anomaly_Detection_Addon.lvlib/Interpolation_Selector.ctl" = enum16{"Nearest", "Bi-Linear"}
  T11 = typedef "DeepLTK_Anomaly_Detection_Addon.lvlib/NN_Paths.ctl" = cluster{"CFG":path, "BIN":path}
  T12 = typedef "DeepLTK_Anomaly_Detection_Addon.lvlib/NNPC_Coreset_Params.ctl" = cluster{"CoreSet_Size":sgl, "Start_idx":i32}
  T13 = typedef "DeepLTK_Anomaly_Detection_Addon.lvlib/NNPC_Setup.ctl" = cluster{"Input_Dims":T14, "mBatch":i32, "Device":T15, "GPU Id":i32}
  T14 = typedef "Deep_Learning_Toolkit_by_Ngene.lvlib/NN_Dims(C,H,W).ctl" = cluster{"C":i32, "H":i32, "W":i32}
  T15 = typedef "Deep_Learning_Toolkit_by_Ngene.lvlib/NN_Device.ctl" = enum16{"CPU", "GPU"}
  T16 = typedef "DeepLTK_Anomaly_Detection_Addon.lvlib/NNPC_Save_CFG.ctl" = cluster{"Add_TimeStamp_SubFolder":bool, "Append_TimeStamp_to_FileNames":bool}
  T17 = typedef "DeepLTK_Anomaly_Detection_Addon.lvlib/NNPC_PreProcessing_Options.ctl" = cluster{"DS_Name":string, "Input_Dims":T14, "Center Crop Size":i32, "Interpolation Type":u32, "Multi-Stage_DownSample?":bool, "Dataset_Stats":T18}
  T18 = typedef "DeepLTK_Anomaly_Detection_Addon.lvlib/NNPC_DS_Stats.ctl" = cluster{"means":T19, "stds":T19}
  T19 = typedef "DeepLTK_Anomaly_Detection_Addon.lvlib/Image_Stats_RGB.ctl" = cluster{"R":sgl, "G":sgl, "B":sgl}
  T20 = typedef "Read_Options.ctl" = cluster{"Read Bads?":bool, "Read GTs?":bool, "Update. DS Stats?":bool}
  T21 = typedef "Deep_Learning_Toolkit_by_Ngene.lvlib/NN_DataSet(In3D_Out3D).ctl" = cluster{"Dataset_Size":i32, "Dims_In":T14, "Labels":string[], "File Paths":path[], "Outputs Ref.":T22, "Inputs Ref.":variant, "Dims_Out":T14}
  T22 = typedef "Deep_Learning_Toolkit_by_Ngene.lvlib/NN_Data_ref(4D_SGL).ctl" = refnum<data-value>
  T23 = typedef "DeepLTK_Anomaly_Detection_Addon.lvlib/NNPC_Instance.ctl" = cluster{"NN":T24, "MemBank_Data":T39, "Name":string}
  T24 = typedef "Deep_Learning_Toolkit_by_Ngene.lvlib/NN.ctl" = cluster{"Name":string, "No of Layers":i32, "mBatch":i32, "Layers":T25[], "Dimty":T26, "Dims_In":T14, "Dims_Out":T14, "Working_Dir":path, "Train?":bool, "Train_Params":T27, "LR_Update_Policy":T30, "Session Data":T32, "Ground_truth":T33, "NNg_hdls":T34, "NN_Device":T15, "GPU Id":i32, "Labels":string[], "Receptive Field":T35[], "Loss_Type":T36, "Loss_Cfg_Prms":variant, "NNG_WS":T37}
  T25 = typedef "Deep_Learning_Toolkit_by_Ngene.lvlib/NN_Layer_ref.ctl" = refnum<data-value>
  T26 = typedef "Deep_Learning_Toolkit_by_Ngene.lvlib/NN_In_Out_Dim-ty.ctl" = enum8{"In1D_Out1D", "In3D_Out1D", "In3D_Out3D", "In3D_OutBBox"}
  T27 = typedef "Deep_Learning_Toolkit_by_Ngene.lvlib/NN_Train_Params.ctl" = cluster{"Optimizer":T28, "Beta_1":sgl, "Beta_2":sgl, "Weight Decay(L1)":sgl, "Weight Decay(L2)":sgl, "Data_Sampling":T29}
  T28 = typedef "Deep_Learning_Toolkit_by_Ngene.lvlib/NN_Train_Optimizer.ctl" = enum16{"SGD", "Adam", "Adagrad", "Adadelta", "RMSProp", "Nesterov"}
  T29 = typedef "Deep_Learning_Toolkit_by_Ngene.lvlib/NN_Train_Data_Sampling.ctl" = enum16{"Random", "Sequential"}
  T30 = typedef "Deep_Learning_Toolkit_by_Ngene.lvlib/NN_LR_Policy_Cfg.ctl" = cluster{"Policy_Type":T31, "LR0":dbl, "k":sgl, "WarmUp_Policy":enum16{"Step", "Ramp"}, "WarmUp_Iter":i32, "WarmUp_Ratio":sgl}
  T31 = typedef "Deep_Learning_Toolkit_by_Ngene.lvlib/NN_LR_Policy_Type.ctl" = enum16{"Manual", "Step", "Exp", "1/t"}
  T32 = typedef "Deep_Learning_Toolkit_by_Ngene.lvlib/NN_Train_Session_Data.ctl" = cluster{"Epochs":sgl, "Tot_Iter":i32, "LR":sgl, "LR_iter":i32}
  T33 = typedef "Deep_Learning_Toolkit_by_Ngene.lvlib/NN_Ground_truth.ctl" = cluster{"Y":variant}
  T34 = typedef "Deep_Learning_Toolkit_by_Ngene.lvlib/nng_cuda_handles.ctl" = cluster{"cudnn":u64, "cublas":u64, "stream":u64, "curand":u64}
  T35 = typedef "Deep_Learning_Toolkit_by_Ngene.lvlib/NN_Dims(V,H).ctl" = cluster{"V":i32, "H":i32}
  T36 = typedef "Deep_Learning_Toolkit_by_Ngene.lvlib/NN_Loss_Type.ctl" = enum16{"None", "MSE", "CrossEntropy", "YOLO_v2", "YOLO_v4"}
  T37 = typedef "Deep_Learning_Toolkit_by_Ngene.lvlib/NNG_WS.ctl" = cluster{"NNG_WS_Mem":T38, "Max_WS_Size":i64}
  T38 = typedef "Deep_Learning_Toolkit_by_Ngene.lvlib/NNg_WS_Mem_DVR.ctl" = refnum<data-value>
  T39 = typedef "DeepLTK_Anomaly_Detection_Addon.lvlib/MemBank_and_Norm_Variants.ctl" = cluster{"MemBank":variant, "MemBank Norm":variant}
  T40 = typedef "imagedata.ctl" = cluster{"image type":i32, "image depth":i32, "image":u8[], "mask":u8[], "colors":u32[], "Rectangle":cluster{"left":i16, "top":i16, "right":i16, "bottom":i16}}
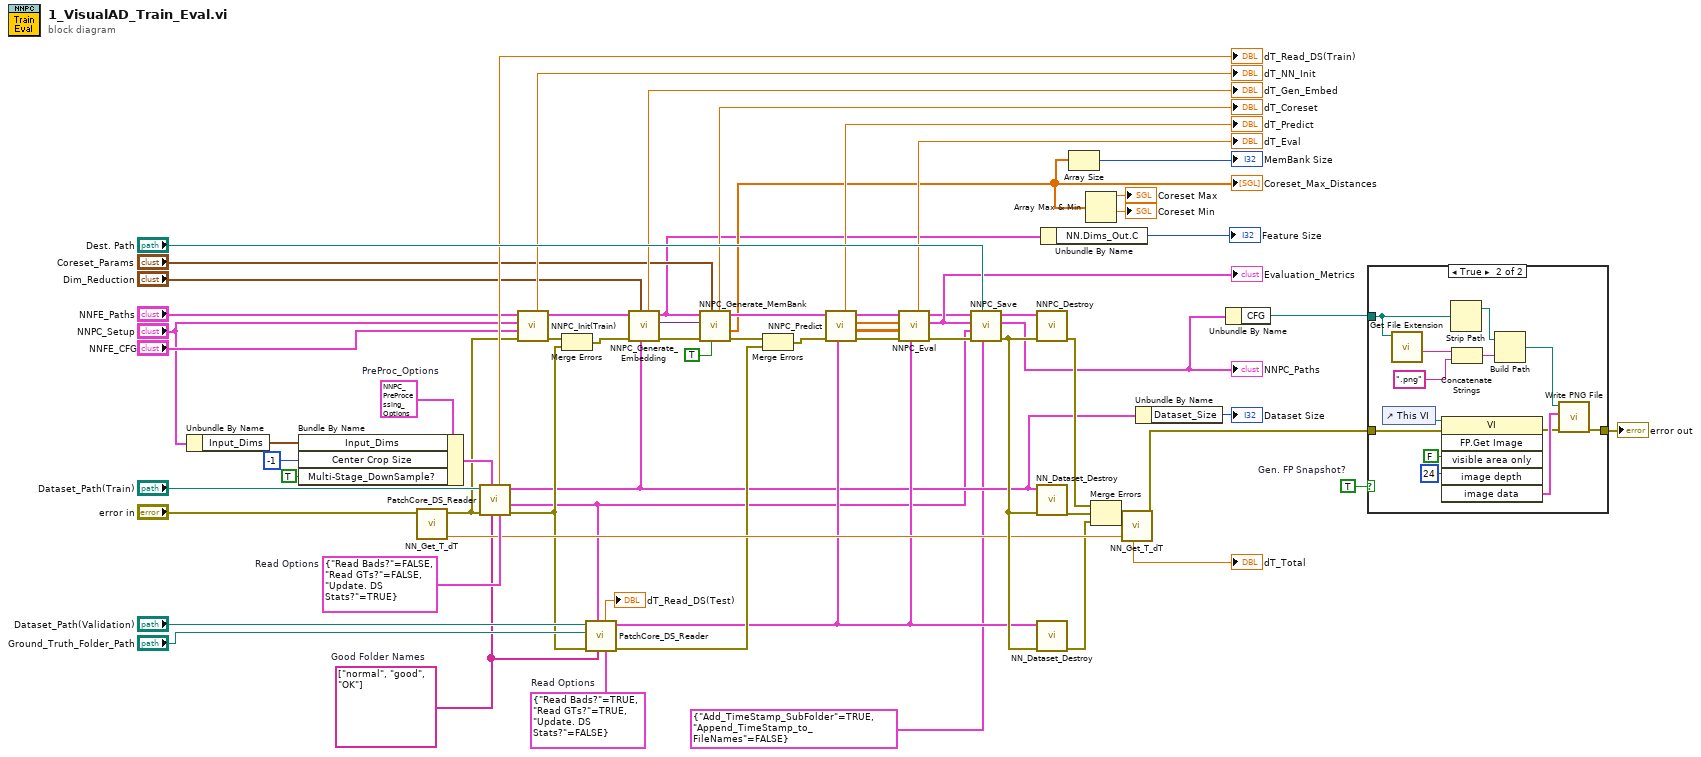
[diagram p0: block diagram]
diagram:
  w4 = T17 {"DS_Name"="", "Input_Dims"={"C"=3, "H"=224, "W"=224}, "Center Crop Size"=0, "Interpolation Type"=1, "Multi-Stage_DownSample?"=FALSE, "Dataset_Stats"={"means"={"R"=0.5385, "G"=0.5348, "B"=0.551}, "stds"={"R"=0.3673, "G"=0.3673, "B"=0.3505}}}  # PreProc_Options
  w21 = TRUE  # Gen. FP Snapshot?
  w49 = T20 {"Read Bads?"=TRUE, "Read GTs?"=TRUE, "Update. DS Stats?"=FALSE}  # Read Options
  w55 = T20 {"Read Bads?"=FALSE, "Read GTs?"=FALSE, "Update. DS Stats?"=TRUE}  # Read Options
  w31 = string[] ["normal", "good", "OK"]  # Good Folder Names
  n1 = Unbundle By Name("NNPC_Setup") -> ("Input_Dims"=w56:T14)
  n2 = Bundle By Name(cluster=w4, "Input_Dims"=w56, "Center Crop Size"=-1, "Multi-Stage_DownSample?"=TRUE) -> (w23:T17)
  n3 = call <vilib>:"NN_Get_T_dT.vi"("error in (no error)"="error in") -> ("T_out"=w53:dbl, "error out"=w12:errorcluster)  [unwired: 6 in, 1 out]
  n4 = call "PatchCore_DS_Reader.vi"("Read Options"=w55, "Good Unique Labels"=w31, "PreProc_Options_in"=w23, "error in (no error)"=w12, "Folder Path"="Dataset_Path(Train)") -> ("error out"=w45:errorcluster, "PreProc_Options_out"=w3:T17, "Dataset"=w24:T21, "dT_DS_Reader"=→"dT_Read_DS(Train)":dbl)  [unwired: 3 in]
  n5 = call <vilib>:"NNPC_Init(Train).vi"("error in"=w12, "NNFE_CFG"="NNFE_CFG", "NNPC_Setup"="NNPC_Setup", "NNFE_Paths"="NNFE_Paths") -> ("error out"=w62:errorcluster, "NNPC_out"=w61:T23, "dT_Init_Train"=→"dT_NN_Init":dbl)  [unwired: 5 in]
  n6 = Merge Errors(w62, w45) -> (w14:errorcluster)
  n7 = call "PatchCore_DS_Reader.vi"("Read Options"=w49, "Good Unique Labels"=w31, "PreProc_Options_in"=w3, "error in (no error)"=w45, "GT Folder Path"="Ground_Truth_Folder_Path", "Folder Path"="Dataset_Path(Validation)") -> ("error out"=w36:errorcluster, "Dataset"=w35:T21, "dT_DS_Reader"=→"dT_Read_DS(Test)":dbl)  [unwired: 2 in, 1 out]
  n8 = call-poly <vilib>:"NNPC_Generate_Embedding.vi"("Dataset"=w24, "Dim_Reduction"="Dim_Reduction", "error in"=w14, "NNPC_in"=w61) -> ("error out"=w13:errorcluster, "Feature_Embeddings"=w15:variant, "NNPC_out"=w6:T23, "dT_Embed"=→"dT_Gen_Embed":dbl)  [unwired: 3 in, 1 out]
  n9 = call <vilib>:"NNPC_Generate_MemBank.vi"("Destroy Embeds Afterwards?"=TRUE, "Coreset_Params"="Coreset_Params", "error in (no error)"=w13, "Feature_Embeddings"=w15, "NNPC_in"=w6) -> ("error out"=w22:errorcluster, "Max_Distances"=w11:sgl[], "NNPC_out"=w39:T23, "dT_Coreset"=→"dT_Coreset":dbl)  [unwired: 3 in]
  "Coreset_Max_Distances" <- w11
  n10 = Merge Errors(w22, w36) -> (w37:errorcluster)
  n11 = call-poly <vilib>:"NNPC_Predict.vi"("Dataset"=w35, "error in (no error)"=w37, "NNPC_in"=w39) -> ("error out"=w40:errorcluster, "Anomaly_Maps"=w42:sgl[][][], "Pred_Scores"=w43:sgl[], "NNPC_out"=w29:T23, "dT_Predict"=→"dT_Predict":dbl)  [unwired: 4 in]
  n12 = call <vilib>:"NNPC_Eval.vi"("Dataset"=w35, "error in (no error)"=w40, "Anomaly_Maps"=w42, "Pred_Scores"=w43, "NNPC_in"=w29) -> ("error out"=w38:errorcluster, "Evaluation_Metrics"=w30:T1, "NNPC_out"=w28:T23, "dT_Eval"=→"dT_Eval":dbl)  [unwired: 3 in]
  "Evaluation_Metrics" <- w30
  n13 = call <vilib>:"NNPC_Save.vi"("Save_Config"=T16 {"Add_TimeStamp_SubFolder"=TRUE, "Append_TimeStamp_to_FileNames"=FALSE}, "Dst_Folder"="Dest. Path", "error in (no error)"=w38, "PreProc_Options_in"=w3, "Evaluation Metrics"=w30, "NNPC_in"=w28) -> ("error out"=w68:errorcluster, "NNPC_Paths"=w20:T11, "NNPC_out"=w7:T23)  [unwired: 3 in]
  "NNPC_Paths" <- w20
  n14 = call <vilib>:"NNPC_Destroy.vi"("error in"=w68, "NNPC_in"=w7) -> ("error out"=w66:errorcluster)  [unwired: 9 in]
  n15 = call-poly <vilib>:"NN_Dataset_Destroy.vi"("error in (no error)"=w68, "Dataset(In3D_Out3D)"=w24) -> ("error out"=w33:errorcluster)  [unwired: 9 in]
  n16 = call-poly <vilib>:"NN_Dataset_Destroy.vi"("error in (no error)"=w68, "Dataset(In3D_Out3D)"=w35) -> ("error out"=w32:errorcluster)  [unwired: 9 in]
  n17 = Unbundle By Name(w6) -> ("NN.Dims_Out.C"=→"Feature Size":i32)
  n18 = Array Size(array=w11) -> (size(s)=→"MemBank Size":i32)
  n19 = Array Max & Min(array=w11) -> (max value=→"Coreset Max":sgl, min value=→"Coreset Min":sgl)  [unwired: 2 out]
  n20 = Merge Errors(w66, w33, w32) -> (w34:errorcluster)
  n21 = call <vilib>:"NN_Get_T_dT.vi"("T_in"=w53, "error in (no error)"=w34) -> ("error out"=w16:errorcluster, "dT"=→"dT_Total":dbl)  [unwired: 5 in, 1 out]
  n22 = Unbundle By Name(w24) -> ("Dataset_Size"=→"Dataset Size":i32)
  n23 = Unbundle By Name(w20) -> ("CFG"=w19:path)
  n24 = case shown="True" w21 {
    tunnel: w19 -> [_ w72]
    tunnel: w16 -> [w69 w71]
    tunnel: [w69 w70] -> w8
    frame False {
    }
    frame True {
      n25 = control-ref of="This VI"() -> (w82:refnum<vi>)
      n26 = call <vilib>:"Get File Extension.vi"("file"=w72) -> ("filename without extension"=w77:string)  [unwired: 6 in, 4 out]
      n27 = invoke class="VI" method="FP.Get Image"(reference=w82, error in=w71, "visible area only"=FALSE ("Visible Area Only"), "image depth"=24 ("Image Depth")) -> (error out=w78:errorcluster, "image data"=w79:T40)  [unwired: 2 in, 4 out]
      n28 = Strip Path(path=w72) -> (stripped path=w74:path)  [unwired: 1 out]
      n29 = Concatenate Strings(w77, ".png" ("string")) -> (w75:string)
      n30 = Build Path(base path=w74, name or relative path=w75) -> (appended path=w73:path)
      n31 = call <vilib>:"Write PNG File.vi"("error in (no error)"=w78, "image data"=w79, "path to PNG file"=w73) -> ("error out"=w70:errorcluster)  [unwired: 7 in, 1 out]
    }
  }
  "error out" <- w8
